vi "Merge.vi"(8 "error in (no error)":errorcluster, 10 "Target":string, 11 "Git Implementation in":refnum<class "Git Implementation.lvclass">) -> (0 "error out":errorcluster, 2 "Status Message":string, 3 "Git Implementation out":refnum<class "Git Implementation.lvclass">)   [LabVIEW 2017, in "Git-LabVIEW.lvlib" / "Git Implementation.lvclass"]
doc: "Carry out a \"git merge\" operation using the behaviour of the Merge-Delegate class contained within this class' private data. By default, a \"No-Conflicts\" Merge Delegate is used.\nGit merge is the second half of a \"git pull\" operation."
uses:
  Git Implementation.lvclass
  Merge Operations/Interface/Merge-Delegate.lvclass
  Merge Operations/No-Conflicts Merge/No-Conflicts Merge.lvclass
  C:/LabVIEW Sources/GitImplementation/Merge Operations/Interface/Merge-Delegate.lvclass
  Git Implementation.lvclass/Git Implementation.ctl
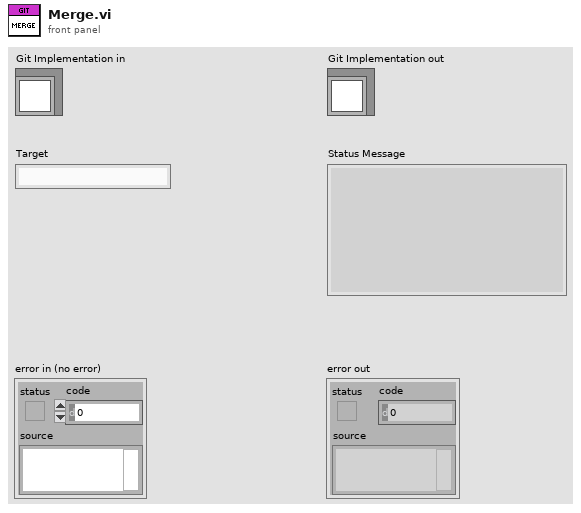
[diagram p1: front panel]
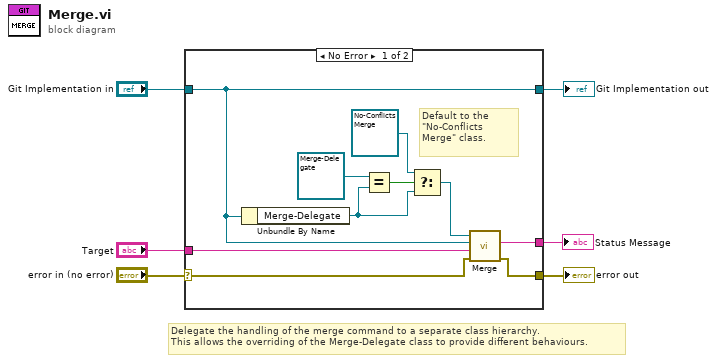
[diagram p0: block diagram]
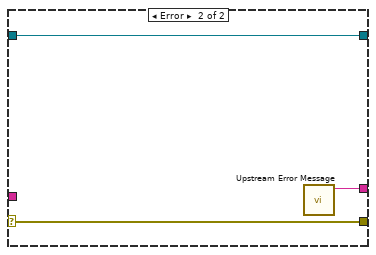
[diagram p2: hidden frame]
diagram:
  # "Delegate the handling of the merge command to a separate class hierarchy.\nThis allows the overriding of the Merge-Delegate class to provide different behaviours."
  n1 = case shown="No Error" "error in (no error)" {
    selector: "error in (no error)" -> [w15 w19]
    tunnel: [w14 w19] -> w5
    tunnel: [w16 w18] -> w3
    tunnel: "Git Implementation in" -> [w16 w18]
    tunnel: [w13 w17] -> w2
    tunnel: "Target" -> [w12 _]
    frame No Error {
      # "Default to the \"No-Conflicts Merge\" class."
      n2 = Unbundle By Name(w16) -> ("Merge-Delegate"=w9:refnum<class "Merge-Delegate.lvclass">)
      n3 = Equal?(x=refnum<class "Merge-Delegate.lvclass"> refnum, y=w9) -> (x = y?=w10:bool)
      n4 = Select(t=refnum<class "No-Conflicts Merge.lvclass"> refnum ("Git-LabVIEW.lvlib:No-Conflicts Merge.lvclass"), s=w10, f=w9) -> (s? t:f=w8:refnum<class "Merge-Delegate.lvclass">)
      n5 = call-dynamic "Merge.vi"("error in (no error)"=w15, "Target"=w12, "Git Implementation"=w16, "Git-Merger in"=w8) -> ("error out"=w14:errorcluster, "Status Message"=w13:string)  [unwired: 6 in]
    }
    frame Error {
      n6 = call "Upstream Error Message.vi"() -> ("Upstream Error Message"=w17:string)  [unwired: 11 in]
    }
  }
  "error out" <- w5
  "Git Implementation out" <- w3
  "Status Message" <- w2
